vi "DetectorVolts.vi"(9 "Detector":dbl, 10 "Detector +/- readback V":dbl, 11 "Digital in":refnum<vi>) -> (2 "Boolean 2":bool, 3 "Boolean":bool)   [LabVIEW 2014]
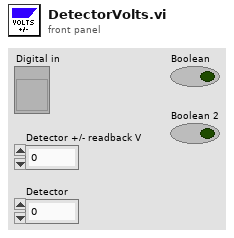
[diagram p1: front panel]
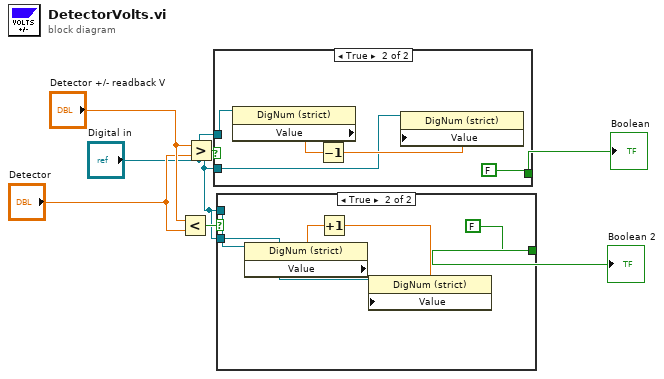
[diagram p0: block diagram]
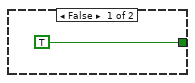
[diagram p2: hidden frame]
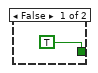
[diagram p3: hidden frame]
diagram:
  n1 = Less?(x="Detector +/- readback V", y="Detector") -> (x < y?=w3:bool)
  n2 = Greater?(x="Detector +/- readback V", y="Detector") -> (0:w2:bool)
  n3 = case shown="True" w2 {
    tunnel: [TRUE FALSE] -> w7
    tunnel: "Digital in" -> [_ w10]
    tunnel: "Digital in" -> [_ w9]
    frame False {
    }
    frame True {
      n4 = property class="DigNum (strict)"(reference=w10) -> ("Value"=w12:dbl)  [unwired: 1 in, 2 out]
      n5 = Decrement(x=w12) -> (x-1=w11:dbl)
      n6 = property class="DigNum (strict)"(reference=w9, "Value"=w11) -> ()  [unwired: 1 in, 2 out]
    }
  }
  "Boolean" <- w7
  n7 = case shown="True" w3 {
    tunnel: [TRUE FALSE] -> w6
    tunnel: "Digital in" -> [_ w16]
    tunnel: "Digital in" -> [_ w15]
    frame False {
    }
    frame True {
      n8 = property class="DigNum (strict)"(reference=w16) -> ("Value"=w18:dbl)  [unwired: 1 in, 2 out]
      n9 = Increment(x=w18) -> (x+1=w17:dbl)
      n10 = property class="DigNum (strict)"(reference=w15, "Value"=w17) -> ()  [unwired: 1 in, 2 out]
    }
  }
  "Boolean 2" <- w6
